vi "racunajec12.vi"() -> ()   [LabVIEW 2014]
uses:
  <vilib>/Analysis/Matrix/Datatypes/RealMatrix.ctl
  <vilib>/Analysis/Matrix/NI_Matrix.lvlib
panel:
  in  "dQ":T1
  in  "Q":T1
  out "ddQ":T1
  in  "T":T1
  in  "g":dbl
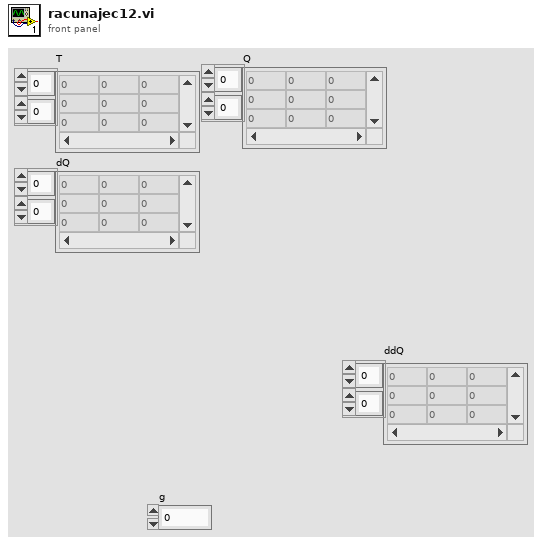
[diagram p1: front panel]
types:
  T1 = typedef "NI_Matrix.lvlib/RealMatrix.ctl" = dbl[][]
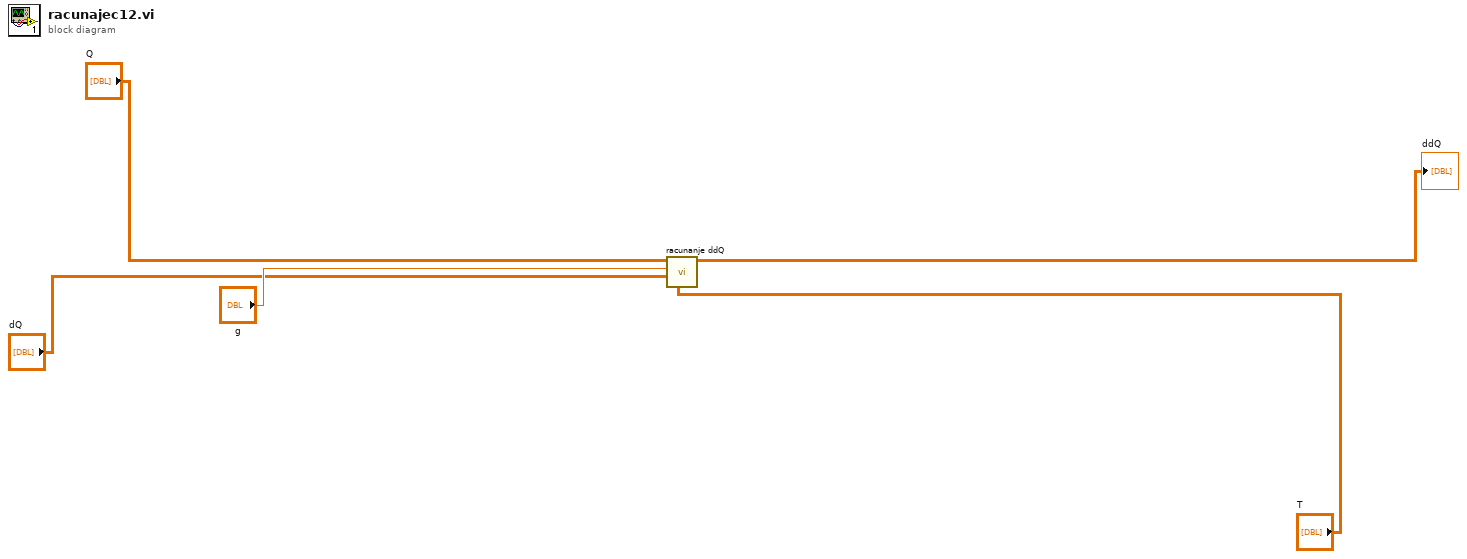
[diagram p0: block diagram]
diagram:
  n1 = call "racunanje ddQ.vi"("T"="T", "dQ"="dQ", "g"="g", "Q"="Q") -> ("ddQ"=→"ddQ":T1)  [unwired: 7 in]
